vi "TCP-IP Link.Set Config.vi"(8 "error in":errorcluster, 10 "TCP-IP Config":T1, 11 "Link Q Name":string="TCP-IP_Link") -> (0 "error out":errorcluster)   [LabVIEW 2024, in "EQMF.lvlib" / "TCP-IP.lvlib"]
uses:
  TCP-IP.lvlib
  Controls/TCP-IP Link.Config.ctl
  Queues/Queue Utils.lvlib
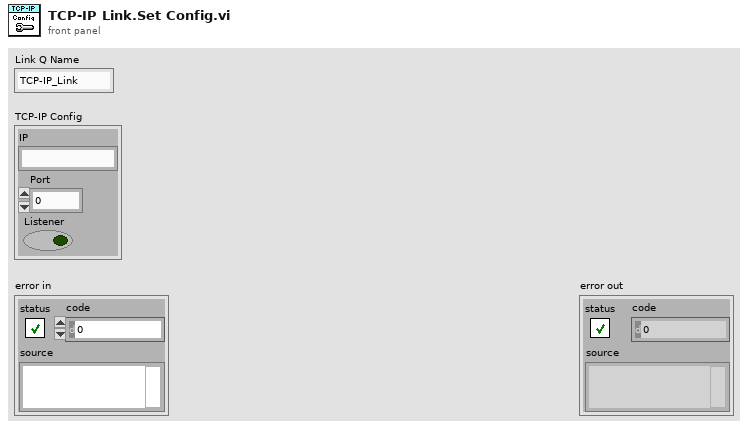
[diagram p1: front panel]
types:
  T1 = typedef "EQMF.lvlib/TCP-IP.lvlib/TCP-IP Link.Config.ctl" = cluster{"IP":string, "Port":u16, "Listener":bool}
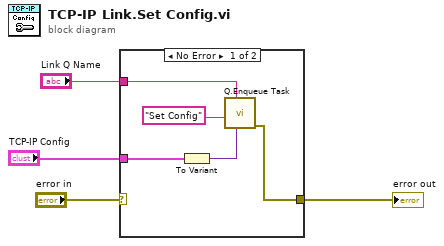
[diagram p0: block diagram]
diagram:
  n1 = case shown="No Error" "error in" {
    selector: "error in" -> [_ w10]
    tunnel: "Link Q Name" -> [w8 _]
    tunnel: [w7 w10] -> w2
    tunnel: "TCP-IP Config" -> [w5 _]
    frame No Error {
      n2 = To Variant(anything=w5) -> (Variant=w6:variant)
      n3 = call "Q.Enqueue Task.vi"("Data1"=w6, "Q Name"=w8, "Task Name"="Set Config") -> ("error out"=w7:errorcluster)  [unwired: 7 in, 1 out]
    }
    frame Error {
    }
  }
  "error out" <- w2
